vi "z_N[Lambda_tau,T,t_0]_Analytical.vi"(6 "t0":ext, 7 "Harmonic f":ext, 8 "N":i32, 10 "T":ext, 11 "tau":ext) -> (3 "z":cxt)   [LabVIEW 2019]
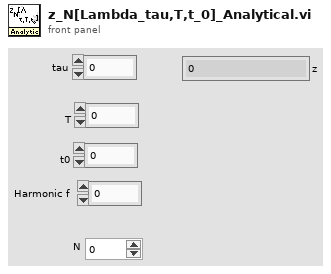
[diagram p1: front panel]
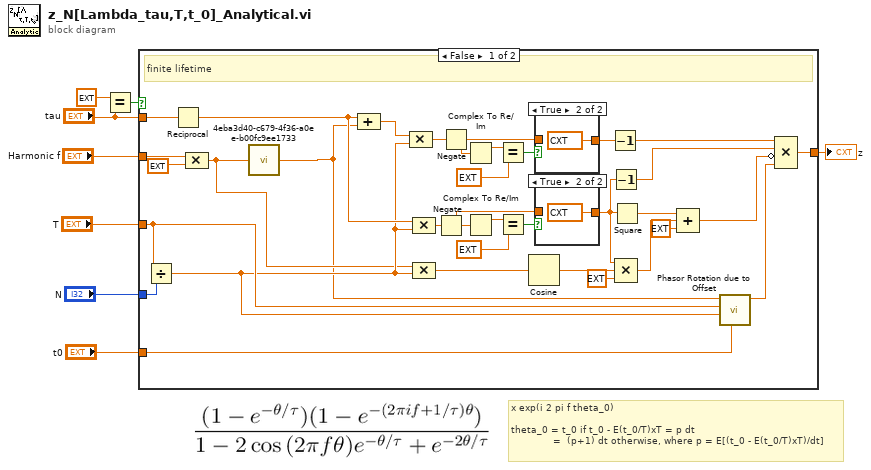
[diagram p0: block diagram]
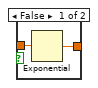
[diagram p2: hidden frame]
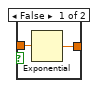
[diagram p3: hidden frame]
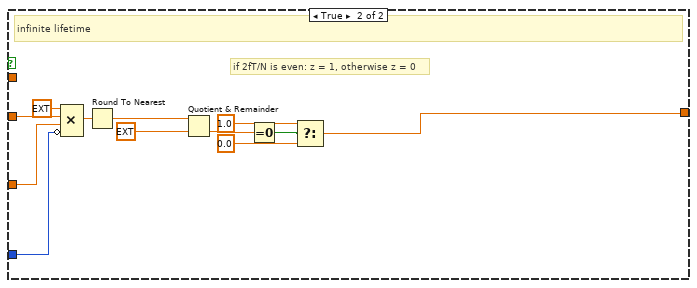
[diagram p4: hidden frame]
diagram:
  # "x exp(i 2 pi f theta_0)\n\ntheta_0 = t_0 if t_0 - E(t_0/T)xT = p dt\n              =  (p+1) dt otherwise, where p = E[(t_0 - E(t_0/T)xT)/dt]"
  n1 = Equal?(x=ext inf, y="tau") -> (x = y?=w1:bool)
  n2 = case shown="False" w1 {
    tunnel: "Harmonic f" -> [w11 w60]
    tunnel: [w38 w51] -> w7
    tunnel: "N" -> [w33 w58]
    tunnel: "T" -> [w25 w59]
    tunnel: "t0" -> [w24 _]
    tunnel: "tau" -> [w12 _]
    frame False {
      # "finite lifetime"
      n3 = Divide(x=w25, y=w33) -> (x/y=w23:ext)
      n4 = Reciprocal(x=w12) -> (1/x=w36:ext)
      n5 = Compound Arithmetic op=MULTIPLY(w11, ext 6.283185307179586477) -> (w10:ext)
      n6 = call "4eba3d40-c679-4f36-a0ee-b00fc9ee1733.vi"("x (1)"=w10) -> ("ix"=w9:cxt)
      n7 = Compound Arithmetic op=ADD(w36, w9) -> (w37:cxt)
      n8 = Compound Arithmetic op=MULTIPLY(w37, w23) -> (w41:cxt)
      n9 = Compound Arithmetic op=MULTIPLY(w36, w23) -> (w35:ext)
      n10 = Compound Arithmetic op=MULTIPLY(w10, w23) -> (w32:ext)
      n11 = Negate(x=w35) -> (-x=w14:ext)
      n12 = Negate(x=w41) -> (-x=w21:cxt)
      n13 = Complex To Re/Im(x + iy=w21) -> (x=w19:ext)  [unwired: 1 out]
      n14 = Complex To Re/Im(x + iy=w14) -> (x=w16:ext)  [unwired: 1 out]
      n15 = Equal?(x=w19, y=ext -inf) -> (x = y?=w18:bool)
      n16 = Equal?(x=w16, y=ext -inf) -> (x = y?=w17:bool)
      n17 = Cosine(x=w32) -> (cos(x)=w31:ext)
      n18 = case shown="True" w18 {
        tunnel: [w47 cxt 0.0+0.0i] -> w40
        tunnel: w21 -> [w46 _]
        frame False {
          n19 = Exponential(1:w46) -> (0:w47:cxt)
        }
        frame True {
        }
      }
      n20 = case shown="True" w17 {
        tunnel: [w44 cxt 0.0+0.0i] -> w13
        tunnel: w14 -> [w43 _]
        frame False {
          n21 = Exponential(1:w43) -> (0:w44:ext)
        }
        frame True {
        }
      }
      n22 = Decrement(x=w40) -> (x-1=w39:cxt)
      n23 = Decrement(x=w13) -> (x-1=w34:cxt)
      n24 = Square(x=w13) -> (x^2=w29:cxt)
      n25 = Compound Arithmetic op=MULTIPLY(w13, w31, ext -2.0 ("value")) -> (w28:cxt)
      n26 = Compound Arithmetic op=ADD(w29, w28, ext 1.0 ("value")) -> (w26:cxt)
      n27 = call "Phasor Rotation due to Offset.vi"("t0"=w24, "dt"=w23, "T"=w25, "j 2 pi f"=w9) -> ("exp(i 2 pi f theta_0)"=w22:cxt)  [unwired: 7 in]
      n28 = Compound Arithmetic op=MULTIPLY(w39, w34, invert w26, w22) -> (w38:cxt)
    }
    frame True {
      # "if 2fT/N is even: z = 1, otherwise z = 0"
      # "infinite lifetime"
      n29 = Compound Arithmetic op=MULTIPLY(ext 2.0 ("value"), w60, w59, invert w58) -> (w56:ext)
      n30 = Round To Nearest(number=w56) -> (nearest integer value=w55:ext)
      n31 = Quotient & Remainder(x=w55, y=ext 2.0) -> (floor(x/y)=w53:ext)  [unwired: 1 out]
      n32 = Equal To 0?(x=w53) -> (x = 0?=w52:bool)
      n33 = Select(t=1.0, s=w52, f=0.0) -> (s? t:f=w51:dbl)
    }
  }
  "z" <- w7
